vi "Append Graph from TDMS to Word Bookmark.vi"(0 "report in":refnum<class "NI_report.lvclass">, 1 "bookmark name (\"\")":string, 5 "data source file path (*.tdms)":path, 7 "group name":string, 9 "channel name(s)":string[](array[string]), 11 "error in (no error)":errorcluster, 13 "graph title (\"\")":string, 14 "graph size (5, 5)":cluster{"height":i32, "width":i32}={"height"=5, "width"=7}) -> (4 "report out":refnum<class "NI_report.lvclass">, 15 "error out":errorcluster)   [LabVIEW 2018, in "WordReportGeneration.lvlib" / "Word_Report.lvclass"]
uses:
  Word_Report.lvclass
  <vilib>/Utility/NIReport.llb/NI_report.lvclass
  <vilib>/Utility/NIReport.llb/Word/NI_Word.lvclass
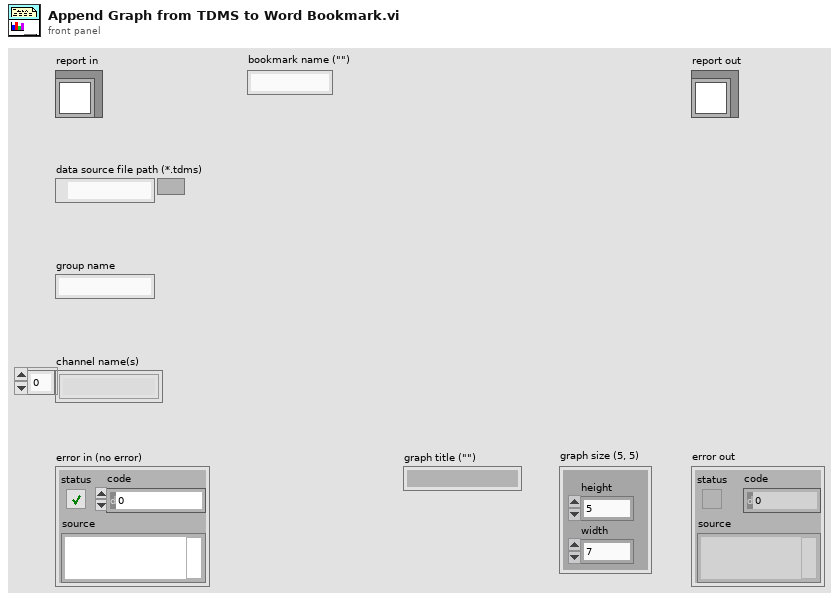
[diagram p1: front panel]
types:
  T1 = enum16{"open", "open or create", "create or replace", "create", "open (read-only)"}
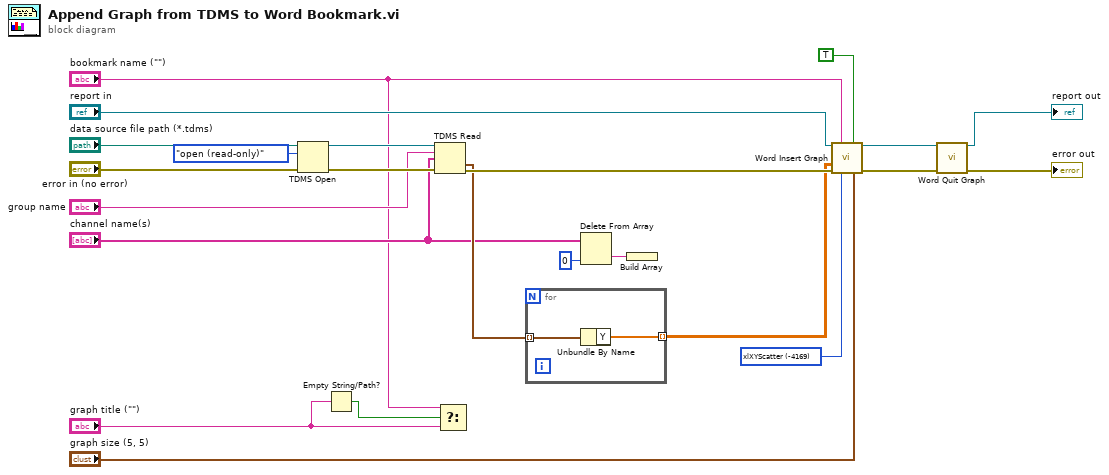
[diagram p0: block diagram]
diagram:
  w10 = -4169 items=["xlColumnClustered"=51, "xlColumnStacked"=52, "xlColumnStacked100"=53, "xl3DColumnClustered"=54, "xl3DColumnStacked"=55, "xl3DColumnStacked100"=56, "xlBarClustered"=57, "xlBarStacked"=58, "xlBarStacked100"=59, "xl3DBarClustered"=60, "xl3DBarStacked"=61, "xl3DBarStacked100"=62, "xlLineStacked"=63, "xlLineStacked100"=64, "xlLineMarkers"=65, "xlLineMarkersStacked"=66, "xlLineMarkersStacked100"=67, "xlPieOfPie"=68, "xlPieExploded"=69, "xl3DPieExploded"=70, "xlBarOfPie"=71, "xlXYScatterSmooth"=72, "xlXYScatterSmoothNoMarkers"=73, "xlXYScatterLines"=74, "xlXYScatterLinesNoMarkers"=75, "xlAreaStacked"=76, "xlAreaStacked100"=77, "xl3DAreaStacked"=78, "xl3DAreaStacked100"=79, "xlDoughnutExploded"=80, "xlRadarMarkers"=81, "xlRadarFilled"=82, "xlSurface"=83, "xlSurfaceWireframe"=84, "xlSurfaceTopView"=85, "xlSurfaceTopViewWireframe"=86, "xlBubble"=15, "xlBubble3DEffect"=87, "xlStockHLC"=88, "xlStockOHLC"=89, "xlStockVHLC"=90, "xlStockVOHLC"=91, "xlCylinderColClustered"=92, "xlCylinderColStacked"=93, "xlCylinderColStacked100"=94, "xlCylinderBarClustered"=95, "xlCylinderBarStacked"=96, "xlCylinderBarStacked100"=97, "xlCylinderCol"=98, "xlConeColClustered"=99, "xlConeColStacked"=100, "xlConeColStacked100"=101, "xlConeBarClustered"=102, "xlConeBarStacked"=103, "xlConeBarStacked100"=104, "xlConeCol"=105, "xlPyramidColClustered"=106, "xlPyramidColStacked"=107, "xlPyramidColStacked100"=108, "xlPyramidBarClustered"=109, "xlPyramidBarStacked"=110, "xlPyramidBarStacked100"=111, "xlPyramidCol"=112, "xl3DColumn"=-4100, "xlLine"=4, "xl3DLine"=-4101, "xl3DPie"=-4102, "xlPie"=5, "xlXYScatter"=-4169, "xl3DArea"=-4098, "xlArea"=1, "xlDoughnut"=-4120, "xlRadar"=-4151] ("graph type (col clustered)")
  n1 = TDMS Open(8:"error in (no error)", 10:T1."open (read-only)" ("operation (0:open)"), 11:"data source file path (*.tdms)") -> (0:w20:errorcluster, 3:w21:refnum<k34>)  [unwired: 4 in]
  n2 = Empty String/Path?(string/path="graph title (\"\")") -> (empty?=w3:bool)
  n3 = TDMS Read(0:w21, 5:"group name", 7:"channel name(s)", 11:w20) -> (10:w17:waveform(dbl)[], 15:w19:errorcluster)  [unwired: 4 in, 4 out]
  n4 = Select(t="bookmark name (\"\")", s=w3, f="graph title (\"\")") -> ()  [unwired: 1 out]
  n5 = for {
    tunnel: w17 -> [w25] mode=indexing
    tunnel: [w24] -> w16 mode=indexing
    n6 = Unbundle By Name(w25) -> ("Y"=w24:dbl[])
  }
  n7 = Delete From Array(array="channel name(s)", index=0) -> (deleted portion=w11:string)  [unwired: 1 in, 1 out]
  n8 = Build Array(w11) -> ()  [unwired: 1 out]
  n9 = call <vilib>:"Word Insert Graph.vi"("report in"="report in", "bookmark name (\"\")"="bookmark name (\"\")", "has legend? (F)"=TRUE, "data"=w16, "error in (no error)"=w19, "graph type (col clustered)"=w10, "graph size (5, 5)"="graph size (5, 5)") -> ("report out"=w8:refnum<class "NI_report.lvclass">, "error out"=w7:errorcluster)  [unwired: 5 in, 2 out]
  n10 = call <vilib>:"Word Quit Graph.vi"("report in"=w8, "error in (no error)"=w7) -> ("report out"=→"report out":refnum<class "NI_report.lvclass">, "error out"=→"error out":errorcluster)  [unwired: 12 in]
